vi "Main.vi"(8 "error in (no error)":errorcluster, 11 "MeritFactor":refnum<class "MeritFactor.lvclass">) -> (0 "error out":errorcluster, 3 "component":refnum<class "MeritFactor.lvclass">)   [LabVIEW 2012, in "MeritFactor.lvclass"]
doc: "Main VI of the component."
uses:
  MeritFactor.lvclass
  <vilib>/Distrio/Murmex/Murmex/command_enum.ctl
  merit factor type.ctl
  MeritFactor.lvclass/MeritFactor.ctl
  <vilib>/Distrio/Murmex/InitialiseMessage/InitialiseMessage.lvclass
  <vilib>/Distrio/Murmex/TerminateMessage/TerminateMessage.lvclass
  <vilib>/Distrio/Murmex/ConfigureMessage/ConfigureMessage.lvclass
  <vilib>/Distrio/Murmex/Murmex/update_cluster.ctl
  <vilib>/Distrio/Murmex/Murmex/Set configure at initialise.vi
  <vilib>/Distrio/Murmex/Murmex/Set log reference.vi
  <vilib>/Distrio/Murmex/Murmex/Set VI reference.vi
  <vilib>/Distrio/Murmex/Murmex/Get ID.vi
  <vilib>/Distrio/Murmex/Murmex/Murmex.lvclass
  <vilib>/Distrio/Murmex/Message/Message.lvclass
panel:
  in  "button::configure":bool
  in  "button::quit":bool
  out "terminate?":bool
  in  "Tab Control":enum32{"User", "Debug"}(tab)
  out "Delta time (ms)":dbl
  in  "Threshold":sgl min=0 max=100
  out "Image maximum":sgl
  out "Image minimum":sgl
  out "Merit factor":dbl
  in  "Brightest bins":dbl min=0.0 max=100.0
  out "Average Image":sgl
  out "STD Image":sgl
  out "SNR Image":sgl
  out "Merit factor type":T1
  out "Image histogram":u32[](graph)
  in  "component ID":string="MF"
  in  "command":T2
  in  "generic command":string
  out "log":string
  in  "button::send":bool
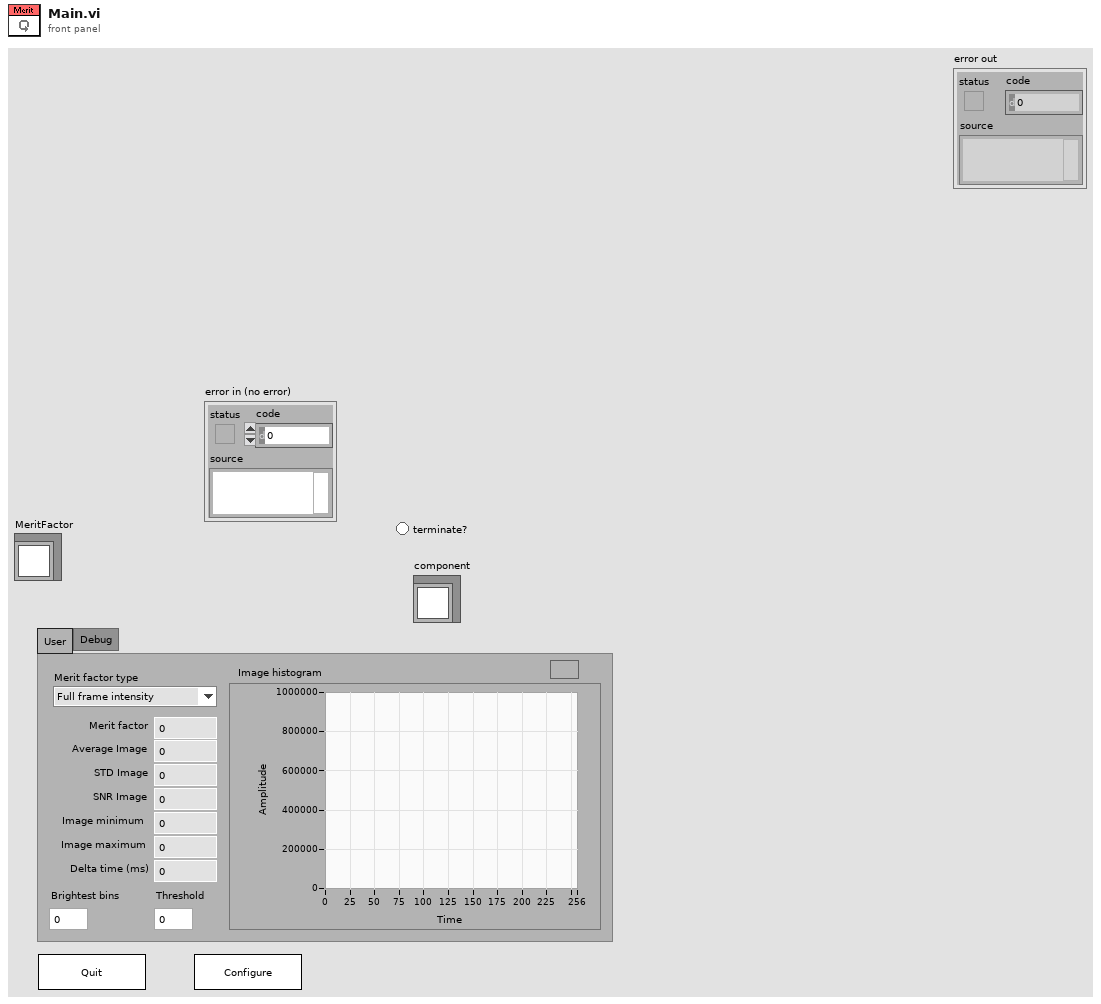
[diagram p1: front panel]
types:
  T1 = typedef "MeritFactor.lvclass/merit factor type.ctl" = enum16{"Full frame intensity", "Brightest pixels intensity", "Contrast (Keller & Stelzer)", "Contrast", "Above-threshold average"}
  T2 = typedef "Murmex.lvlib/Murmex.lvclass/command_enum.ctl" = enum16{"null", "initialise", "reset", "terminate", "acknowledge", "update", "inspect", "inform", "proceed", "start", "stop", "fetch", "configure", "generic"}
  T3 = enum8{"Enabled", "Disabled", "Disabled and Grayed Out"}
  T4 = typedef "Murmex.lvlib/Murmex.lvclass/update_cluster.ctl" = cluster{"target ID":string, "key chains":string[], "values":variant[]}
  T5 = typedef "Murmex.lvlib/Murmex.lvclass/Event type enumerations.ctl" = enum16{"before", "after"}
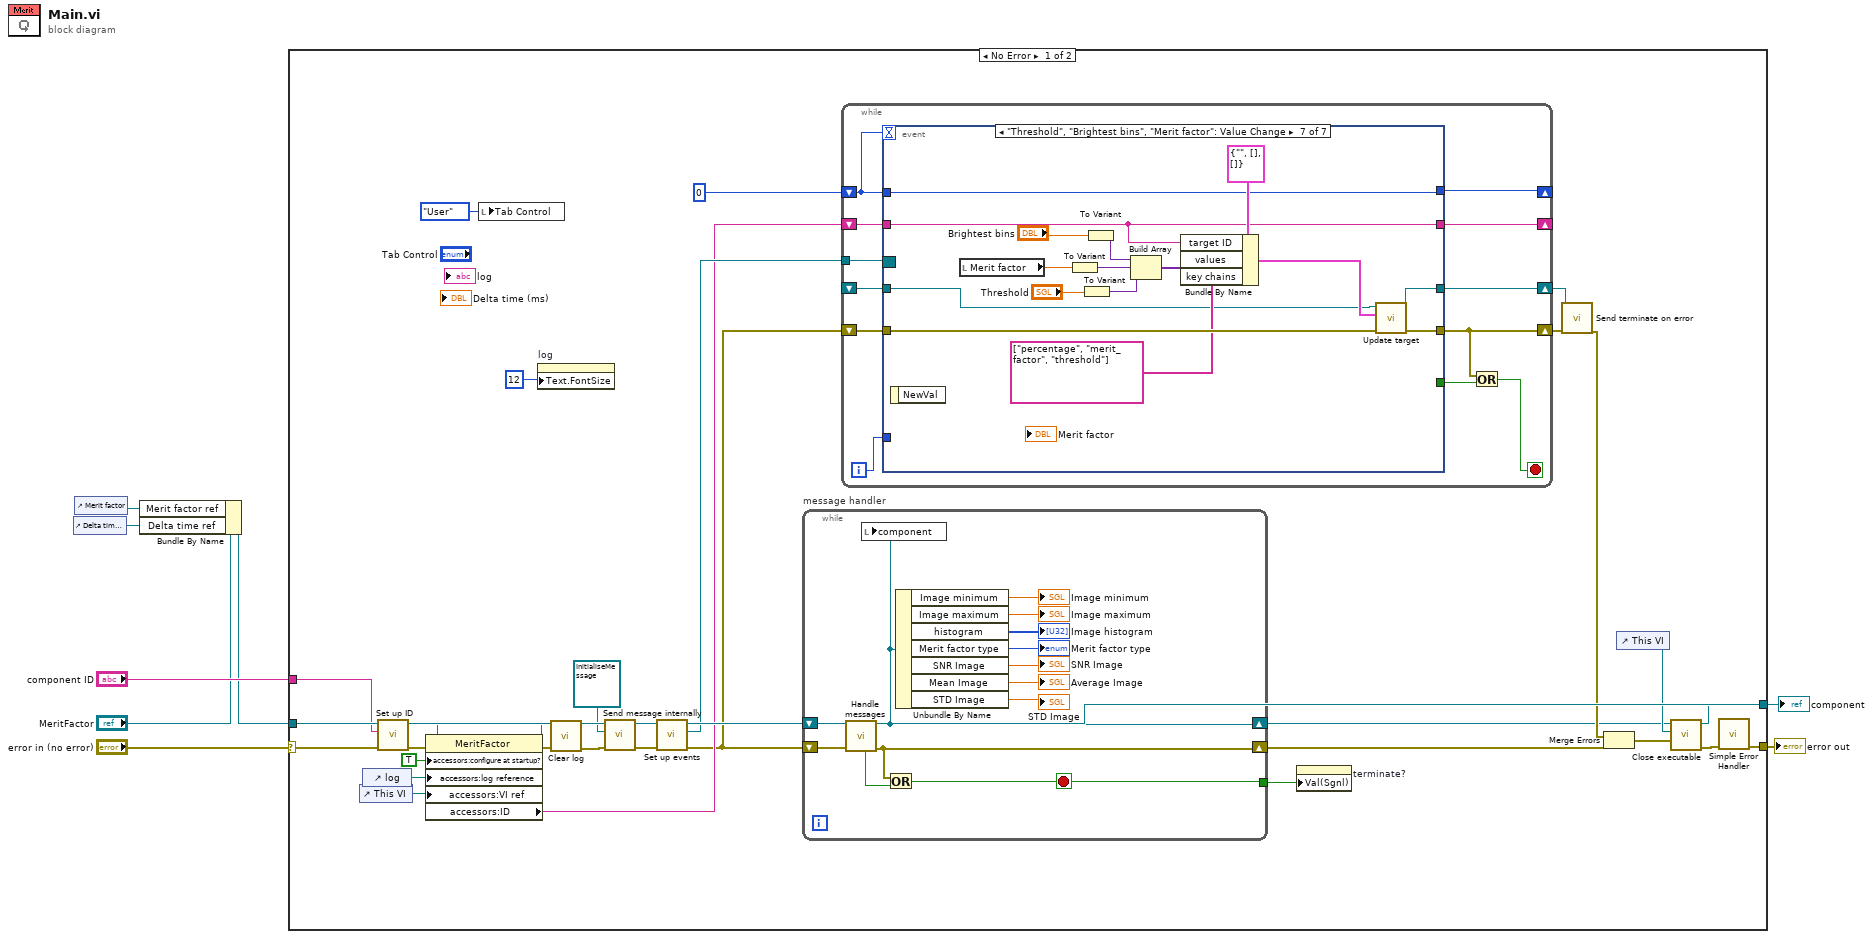
[diagram p0: block diagram]
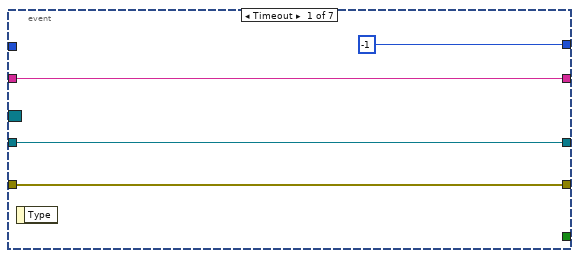
[diagram p2: hidden frame]
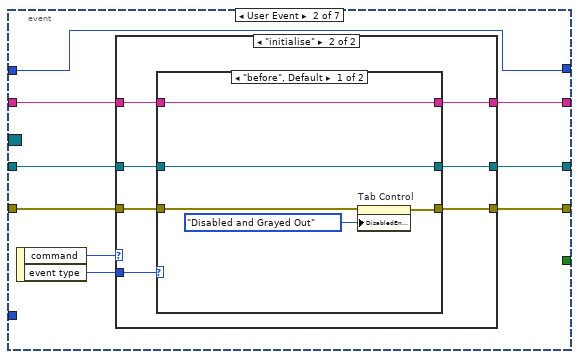
[diagram p3: hidden frame]
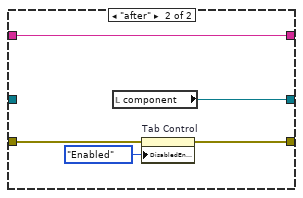
[diagram p5: hidden frame]
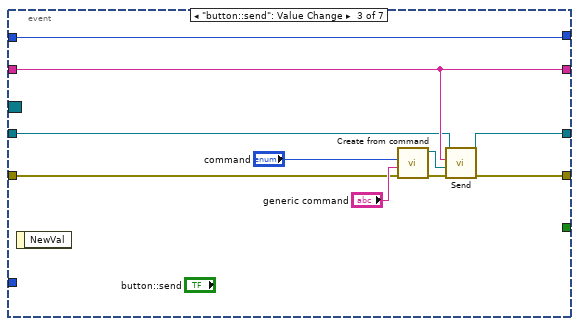
[diagram p6: hidden frame]
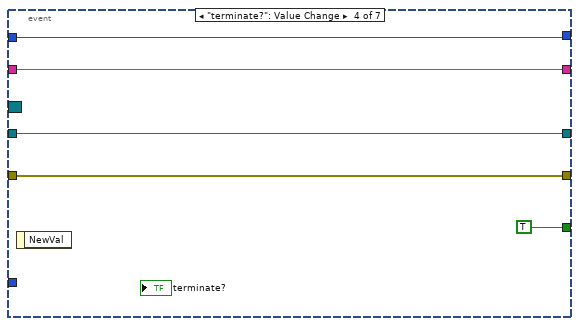
[diagram p7: hidden frame]
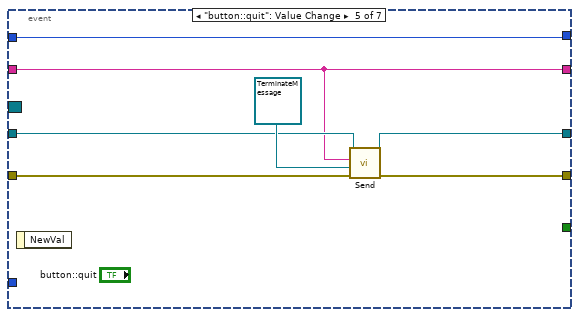
[diagram p8: hidden frame]
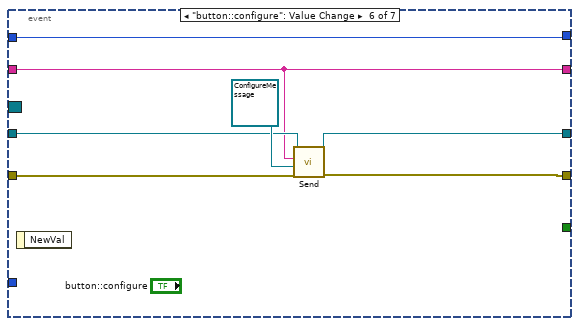
[diagram p9: hidden frame]
diagram:
  n1 = control-ref of="Delta time (ms)"() -> (w1:refnum<vi>)
  n2 = control-ref of="Merit factor"() -> (w2:refnum<vi>)
  n3 = Bundle By Name(cluster="MeritFactor", "Merit factor ref"=w2, "Delta time ref"=w1) -> (w3:refnum<class "MeritFactor.lvclass">)
  "component" <- w3
  n4 = case shown="No Error" "error in (no error)" {
    selector: "error in (no error)" -> [w40 w145]
    tunnel: w3 -> [w39 w144]
    tunnel: "component ID" -> [w38 _]
    tunnel: [w13 w145] -> w5
    tunnel: [w10 w144] -> _
    frame No Error {
      n5 = control-ref of="This VI"() -> (w33:refnum<vi>)
      n6 = control-ref of="log"() -> (w34:refnum<vi>)
      n7 = call <vilib>:"Set up ID.vi"("error in (no error)"=w40, "component ID"=w38, "MurmexBase in"=w39) -> ("error out"=w37:errorcluster, "MurmexBase out"=w36:refnum<class "MeritFactor.lvclass">)  [unwired: 6 in, 1 out]
      n8 = property class="MeritFactor"(reference=w36, error in=w37, "accessors:configure at startup?"=TRUE ("configure at startup?"), "accessors:log reference"=w34, "accessors:VI ref"=w33) -> (reference out=w28:refnum<class "MeritFactor.lvclass">, error out=w32:errorcluster, "accessors:ID"=w22:string)
      n9 = local write "Tab Control"(enum32{"User", "Debug"}."User" ("Tab Control")) -> ()
      n10 = property on="log" class="Str"("Text.FontSize"=u32 12 ("Text.Font:Size")) -> ()  [unwired: 2 in, 2 out]
      n11 = call <vilib>:"Clear log.vi"("error in (no error)"=w32, "MurmexBase in"=w28) -> ("error out"=w30:errorcluster, "MurmexBase out"=w29:refnum<class "MeritFactor.lvclass">)  [unwired: 8 in]
      n12 = call <vilib>:"Send message internally.vi"("error in (no error)"=w30, "Message"=refnum<class "InitialiseMessage.lvclass"> refnum ("Distrio Murmex 1.0:InitialiseMessage"), "Murmex in"=w29) -> ("error out"=w27:errorcluster, "Murmex out"=w26:refnum<class "MeritFactor.lvclass">)  [unwired: 7 in]
      n13 = call <vilib>:"Set up events.vi"("error in (no error)"=w27, "MurmexBase in"=w26) -> ("error out"=w21:errorcluster, "Event Registration Refnum"=w24:refnum<event-registration>, "MurmexBase out"=w25:refnum<class "MeritFactor.lvclass">)  [unwired: 7 in]
      n14 = while "message handler" {
        shift-right: [w140] -> w9
        shift-left: w21 -> [w143]
        shift-right: [w138] -> w14
        shift-left: w25 -> [w142]
        tunnel: [w139] -> w12
        stop <- w139 stop-if-true
        n15 = call <vilib>:"Handle messages.vi"("error in (no error)"=w143, "Murmex in"=w142) -> ("error out"=w140:errorcluster, "Murmex out"=w138:refnum<class "MeritFactor.lvclass">, "terminated?"=w141:bool)  [unwired: 7 in]
        n16 = local write "component"(w138) -> ()
        n17 = Or(x=w140, y=w141) -> (x .or. y?=w139:bool)
        n18 = Unbundle By Name(w138) -> ("Image minimum"=→"Image minimum":sgl, "Image maximum"=→"Image maximum":sgl, "histogram"=→"Image histogram":u32[], "Merit factor type"=→"Merit factor type":T1, "SNR Image"=→"SNR Image":sgl, "Mean Image"=→"Average Image":sgl, "STD Image"=→"STD Image":sgl)
      }
      n19 = while {
        tunnel: w24 -> [w47]
        shift-right: [w51] -> _
        shift-left: 0 -> [w52]
        shift-right: [w49] -> _
        shift-left: w22 -> [w50]
        shift-right: [w46] -> w16
        shift-left: w21 -> [w48]
        shift-right: [w44] -> w15
        shift-left: _ -> [w43]
        i -> [w41]
        stop <- w45 stop-if-true
        n20 = event shown="[6] \"Threshold\", \"Brightest bins\", \"Merit factor\": Value Change" {
          selector: w47 -> [_ _ _ _ _ _ _]
          dyn-events: _ -> [_ _ _ _ _ _ _]
          timeout: w52 -> [_ _ _ _ _ _ _]
          tunnel: w52 -> [_ w57 w95 w100 w101 w108 w122]
          tunnel: [-1 w57 w95 w100 w101 w108 w122] -> w51
          tunnel: w50 -> [w55 w61 w88 w99 w102 w109 w125]
          tunnel: [w55 w60 w88 w99 w102 w109 w125] -> w49
          tunnel: [w54 w58 w90 w97 w106 w113 w128] -> w46
          tunnel: w48 -> [w54 w59 w92 w97 w107 w114 w127]
          tunnel: [w53 w63 w86 w98 w103 w110 w120] -> w44
          tunnel: w43 -> [w53 w62 w87 w98 w104 w111 w121]
          tunnel: [_ _ _ TRUE _ _ _] -> w42
          tunnel: w41 -> [_ _ _ _ _ _ _]
          event Timeout {
            n21 = event-data() -> ()  [unwired: 1 in, 1 out]
          }
          event User Event {
            n22 = event-data() -> ("command"=w65:T2, "event type"=w64:T5)  [unwired: 1 in]
            n23 = case shown="\"initialise\"" w65 {
              tunnel: w64 -> [_ w75]
              tunnel: [w67 w74] -> w63
              tunnel: w62 -> [w67 w73]
              tunnel: w61 -> [w68 w72]
              tunnel: [w68 w71] -> w60
              tunnel: w59 -> [w66 w70]
              tunnel: [w66 w69] -> w58
              frame "null", Default {
              }
              frame "initialise" {
                n24 = case shown="\"before\", Default" w75 {
                  tunnel: [w79 w81] -> w74
                  tunnel: w73 -> [w79 _]
                  tunnel: w72 -> [w80 w85]
                  tunnel: [w80 w85] -> w71
                  tunnel: w70 -> [w78 w84]
                  tunnel: [w77 w83] -> w69
                  frame "before", Default {
                    n25 = property on="Tab Control" class="TabCtl (strict)"(error in=w78, "DisabledEnum"=T3."Disabled and Grayed Out" ("Disabled")) -> (error out=w77:errorcluster)  [unwired: 1 in, 1 out]
                  }
                  frame "after" {
                    n26 = local read "component"() -> (w81:refnum<class "MeritFactor.lvclass">)
                    n27 = property on="Tab Control" class="TabCtl (strict)"(error in=w84, "DisabledEnum"=T3."Enabled" ("Disabled")) -> (error out=w83:errorcluster)  [unwired: 1 in, 1 out]
                  }
                }
              }
            }
          }
          event "button::send": Value Change {
            n28 = event-data() -> ()  [unwired: 1 in, 1 out]
            n29 = call <vilib>:"Create from command.vi"("error in (no error)"=w92, "generic command"="generic command", "command"="command") -> ("error out"=w91:errorcluster, "Message out"=w89:refnum<class "Message.lvclass">)  [unwired: 7 in]
            n30 = call <vilib>:"Send.vi"("error in (no error)"=w91, "Message"=w89, "recipient"=w88, "Murmex in"=w87) -> ("error out"=w90:errorcluster, "Murmex out"=w86:refnum<class "MeritFactor.lvclass">)  [unwired: 6 in]
          }
          event "terminate?": Value Change {
            n31 = event-data() -> ()  [unwired: 1 in, 1 out]
          }
          event "button::quit": Value Change {
            n32 = event-data() -> ()  [unwired: 1 in, 1 out]
            n33 = call <vilib>:"Send.vi"("error in (no error)"=w107, "Message"=refnum<class "TerminateMessage.lvclass"> refnum ("Distrio Murmex 1.0:TerminateMessage"), "recipient"=w102, "Murmex in"=w104) -> ("error out"=w106:errorcluster, "Murmex out"=w103:refnum<class "MeritFactor.lvclass">)  [unwired: 6 in]
          }
          event "button::configure": Value Change {
            n34 = event-data() -> ()  [unwired: 1 in, 1 out]
            n35 = call <vilib>:"Send.vi"("error in (no error)"=w114, "Message"=refnum<class "ConfigureMessage.lvclass"> refnum ("Distrio Murmex 1.0:ConfigureMessage"), "recipient"=w109, "Murmex in"=w111) -> ("error out"=w113:errorcluster, "Murmex out"=w110:refnum<class "MeritFactor.lvclass">)  [unwired: 6 in]
          }
          event "Threshold", "Brightest bins", "Merit factor": Value Change {
            n36 = event-data() -> ()  [unwired: 1 in, 1 out]
            n37 = local read "Merit factor"() -> (w118:dbl)
            n38 = To Variant(anything=w118) -> (Variant=w117:variant)
            n39 = To Variant(anything="Threshold") -> (Variant=w115:variant)
            n40 = To Variant(anything="Brightest bins") -> (Variant=w130:variant)
            n41 = Build Array(w130, w117, w115) -> (w124:variant[])
            n42 = Bundle By Name(cluster=T4 {"target ID"="", "key chains"=[], "values"=[]} ("update cluster"), "target ID"=w125, "values"=w124, "key chains"=string[] ["percentage", "merit_factor", "threshold"]) -> (w129:T4)
            n43 = call <vilib>:"Update target.vi"("error in (no error)"=w127, "update cluster"=w129, "MurmexBase in"=w121) -> ("error out"=w128:errorcluster, "MurmexBase out"=w120:refnum<class "MeritFactor.lvclass">)  [unwired: 7 in]
          }
        }
        n44 = Or(x=w46, y=w42) -> (x .or. y?=w45:bool)
      }
      n45 = property on="terminate?" class="Bool (strict)"("Val(Sgnl)"=w12) -> ()  [unwired: 2 in, 2 out]
      n46 = call <vilib>:"Send terminate on error.vi"("error in (no error)"=w16, "Murmex in"=w15) -> ("error out"=w20:errorcluster)  [unwired: 8 in, 1 out]
      n47 = Merge Errors(w20, w9) -> (w19:errorcluster)
      n48 = control-ref of="This VI"() -> (w18:refnum<vi>)
      n49 = call <vilib>:"Close executable.vi"("error in (no error)"=w19, "main VI ref (optional)"=w18, "MurmexBase in"=w14) -> ("error out"=w17:errorcluster, "MurmexBase out"=w10:refnum<class "MeritFactor.lvclass">)  [unwired: 7 in]
      n50 = call <vilib>:"Simple Error Handler.vi"("error in (no error)"=w17) -> ("error out"=w13:errorcluster)  [unwired: 4 in, 4 out]
    }
    frame Error {
    }
  }
  "error out" <- w5
